vi "TrianglesMaxMin.vi"(11 "Triangles":T2[](array[typedef])) -> (1 "Center":T1, 2 "MaxDims":T1, 3 "MinDims":T1)   [LabVIEW 2014]
uses:
  TypeDefs/TriangleFace.ctl
  TypeDefs/Point3D.ctl
  <vilib>/Analysis/baseanly.llb/Mean (DBL).vi
  <vilib>/Analysis/NI_AALBase.lvlib
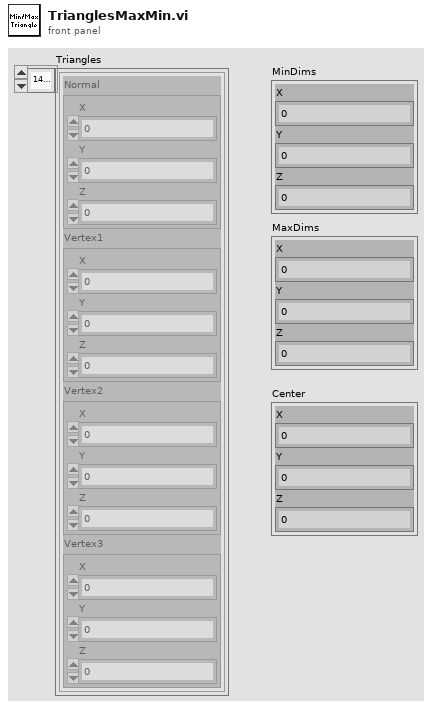
[diagram p1: front panel]
types:
  T1 = typedef "Point3D.ctl" = cluster{"X":sgl, "Y":sgl, "Z":sgl}
  T2 = typedef "TriangleFace.ctl" = cluster{"Normal":T1, "Vertex1":T1, "Vertex2":T1, "Vertex3":T1}
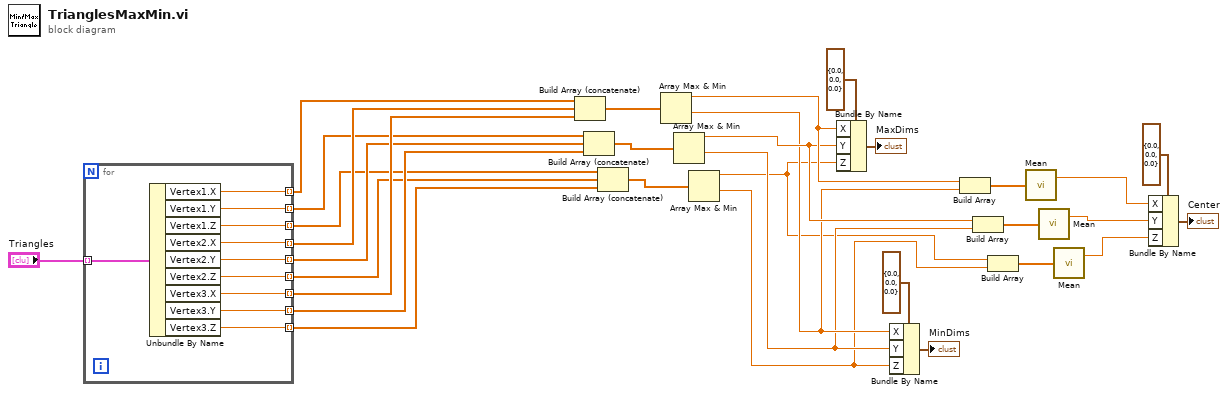
[diagram p0: block diagram]
diagram:
  n1 = for {
    tunnel: "Triangles" -> [w41] mode=indexing
    tunnel: [w40] -> w15 mode=indexing
    tunnel: [w39] -> w11 mode=indexing
    tunnel: [w38] -> w8 mode=indexing
    tunnel: [w37] -> w14 mode=indexing
    tunnel: [w36] -> w10 mode=indexing
    tunnel: [w35] -> w7 mode=indexing
    tunnel: [w34] -> w13 mode=indexing
    tunnel: [w33] -> w9 mode=indexing
    tunnel: [w32] -> w6 mode=indexing
    n2 = Unbundle By Name(w41) -> ("Vertex1.X"=w40:sgl, "Vertex1.Y"=w39:sgl, "Vertex1.Z"=w38:sgl, "Vertex2.X"=w37:sgl, "Vertex2.Y"=w36:sgl, "Vertex2.Z"=w35:sgl, "Vertex3.X"=w34:sgl, "Vertex3.Y"=w33:sgl, "Vertex3.Z"=w32:sgl)
  }
  n3 = Build Array (concatenate)(w15, w14, w13) -> (w31:sgl[])
  n4 = Build Array (concatenate)(w11, w10, w9) -> (w30:sgl[])
  n5 = Build Array (concatenate)(w8, w7, w6) -> (w12:sgl[])
  n6 = Array Max & Min(array=w31) -> (max value=w25:sgl, min value=w5:sgl)  [unwired: 2 out]
  n7 = Array Max & Min(array=w30) -> (max value=w22:sgl, min value=w4:sgl)  [unwired: 2 out]
  n8 = Array Max & Min(array=w12) -> (max value=w3:sgl, min value=w2:sgl)  [unwired: 2 out]
  n9 = Bundle By Name(cluster=T1 {"X"=0.0, "Y"=0.0, "Z"=0.0} ("Point3D"), "X"=w25, "Y"=w22, "Z"=w3) -> (→"MaxDims":T1)
  n10 = Bundle By Name(cluster=T1 {"X"=0.0, "Y"=0.0, "Z"=0.0} ("Point3D"), "X"=w5, "Y"=w4, "Z"=w2) -> (→"MinDims":T1)
  n11 = Build Array(w25, w5) -> (w24:sgl[])
  n12 = Build Array(w22, w4) -> (w23:sgl[])
  n13 = Build Array(w3, w2) -> (w1:sgl[])
  n14 = call-poly <vilib>:"Mean.vi"("X"=w24) -> ("mean"=w19:dbl)  [unwired: 1 out]
  n15 = call-poly <vilib>:"Mean.vi"("X"=w23) -> ("mean"=w18:dbl)  [unwired: 1 out]
  n16 = call-poly <vilib>:"Mean.vi"("X"=w1) -> ("mean"=w17:dbl)  [unwired: 1 out]
  n17 = Bundle By Name(cluster=T1 {"X"=0.0, "Y"=0.0, "Z"=0.0} ("Point3D"), "X"=w19, "Y"=w18, "Z"=w17) -> (→"Center":T1)
